vi "Write File+ (string).vi"(4 "convert eol? (no:F)":bool caption="EOL konvertieren? (no:F)", 5 "string":string caption="String", 6 "error in (no error)":errorcluster caption="Fehler (Eingang, kein Fehler)", 7 "pos offset (bytes:0)":i32 caption="Pos.-Offset (Bytes:0)", 8 "pos mode (rel. to end:1)":enum16{"start", "end", "current"}(ring)=enum."end" caption="Pos.-Modus (relativ zum Ende:1)", 9 "refnum":refnum<file> caption="RefNum") -> (0 "error out":errorcluster caption="Fehler (Ausgang)", 1 "mark after write (bytes)":i32 caption="Dateimarke nach Schreibvorgang (Zeichen)", 3 "dup refnum":refnum<file> caption="RefNum (Kopie)")   [LabVIEW 2009]
doc: "Schreibt in die angegebenen Stelle einen String aus einer Byte-Stream-Datei; der voreingestellte Platz ist das Ende der Datei. Das VI überprüft eingehende und interne Fehler und schreibt nicht, wenn ein Eingangsfehler auftritt.\n\n'RefNum' ist die Referenz zur geöffneten Datei.\n\n'Pos.-Modus' legt fest, an welcher Stelle, relativ zu 'Pos.-Offset', zu schreiben begonnen wird:\n\n 0: am Anfang der Datei plus Pos.-Offest.\n\n 1: am Ende der Datei plus Pos.-Offest. Dies ist die Standardeinstellung.\n\n 2: an der aktuellen Markierung plus Pos.-Offset.\n\n'Pos.-Offset' legt in Zeichen fest, wie weit entfernt von 'Pos.-Modus' begonnen wird. Der Standardwert ist 0.\n\nZeichen-String enthält die Daten, die das VI in die Datei schreibt.\n\nEOL konvertieren? konvertiert das LabVIEW-spezifische Zeilenende (EOL) in die plattformspezifische Zeilenendemarkierung, falls die Option auf TRUE gesetzt ist. Führt bei FALSE (Standardwert) keine Aktion aus.\n\nFehlereingang ist ein Cluster mit 3 Elementen (Fehler?, Code, und Quelle), das den bisherigen Fehlerstatus beschreibt, wenn bei vorher ausgeführten VIs ein Fehler aufgetreten ist. Das VI kann nur dann normal ausgeführt werden, wenn kein Eingangsfehler vorliegt; sonst wird der vorher aufgetretene Fehler weitergeleitet. Fehler? ist TRUE, wenn ein Fehler aufgetreten ist; die Voreinstellung ist FALSE. Code ist der Fehlercode; die Voreinstellung ist 0. Quelle ist in den meisten Fällen der Name des VIs oder der Funktion in welcher der Fehler aufgetreten ist; die Voreinstellung ist ein leerer String. \n\nRefNum (Kopie) leitet die Referenznummer weiter.\n\nDie Dateimarke zeigt nach dem Schreiben auf die nächste Postion nach dem letzten geschriebenen Zeichen.\n\nFehlerausgang ist ein Cluster mit 3 Elementen (Fehler?, Code, und Quelle) welches den Fehlerstatus nach Ablauf des VIs beschreibt. Wenn kein Eingangsfehler auftrat, wird das VI normal ausgeführt und der Fehlerausgang enthält den Fehlerstatus dieses VIs; wenn ein Eingangsfehler auftrat wird diesen an den Fehlerausgang weitergegeben."
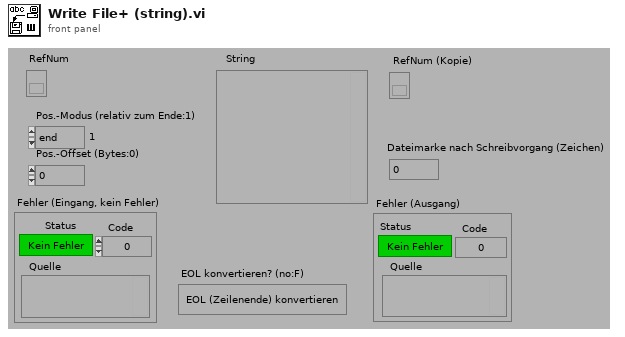
[diagram p1: front panel]
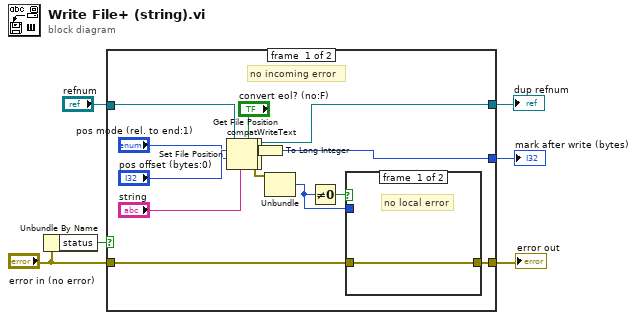
[diagram p0: block diagram]
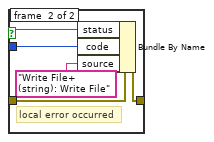
[diagram p2: hidden frame]
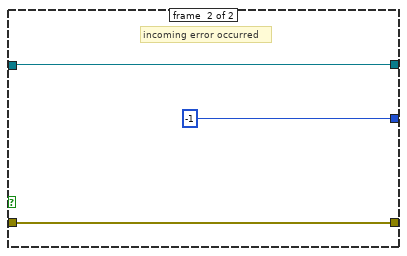
[diagram p3: hidden frame]
diagram:
  n1 = Unbundle By Name("error in (no error)") -> ("status"=w6:bool)
  n2 = case shown="False" w6 {
    tunnel: [w16 w31] -> w5
    tunnel: [w21 -1] -> w4
    tunnel: [w20 w30] -> w3
    tunnel: "refnum" -> [w19 w30]
    tunnel: "error in (no error)" -> [w15 w31]
    frame #0 {
      # "no incoming error"
      n3 = Set File Position(offset (in bytes) (0)="pos offset (bytes:0)", refnum=w19, from (0:start)="pos mode (rel. to end:1)") -> (refnum out=w11:refnum<file>, error out=w10:errorcluster)  [unwired: 1 in]
      n4 = call <vilib>:"compatWriteText.vi"("convert eol (F)"="convert eol? (no:F)", "data"="string", "error in"=w10, "refnum"=w11) -> ("error out"=w8:errorcluster, "dup refnum"=w9:refnum<file>)  [unwired: 6 in]
      n5 = Get File Position(4:w8, 7:w9) -> (0:w17:errorcluster, 2:w7:i64, 3:w20:refnum<file>)
      n6 = To Long Integer(number=w7) -> (32bit integer=w21:i32)
      n7 = Unbundle(w17) -> ("code"=w13:i32)  [unwired: 2 out]
      n8 = Not Equal To 0?(x=w13) -> (x != 0?=w14:bool)
      n9 = case shown="True" w14 {
        selector: w14 -> [_ w25]
        tunnel: w13 -> [_ w28]
        tunnel: [w24 w26] -> w16
        tunnel: w15 -> [w24 w27]
        frame #0 {
          # "no local error"
        }
        frame #1 {
          # "local error occurred"
          n10 = Bundle By Name(cluster=w27, "status"=w25, "code"=w28, "source"="Write File+ (string): Write File") -> (w26:errorcluster)
        }
      }
    }
    frame #1 {
      # "incoming error occurred"
    }
  }
  "error out" <- w5
  "mark after write (bytes)" <- w4
  "dup refnum" <- w3
